vi "OEE_SCREEN_2_line_performance_into_cluster.vi"(6 "SCREEN_2":T1={"header_part_no"="-", "header_customer"="-", "performance_percentage"="-", "performance_target"="-", "performance_actual"="-", "performance_header"="PERFORMANCE", "performance_target_header"="TARGET", "performance_actual_header"="ACTUAL", "screen_2_header"=""}, 11 "hourly_ok_count":string[][](array[string])) -> (4 "SCREEN_2":T1={"header_part_no"="-", "header_customer"="-", "performance_percentage"="-", "performance_target"="-", "performance_actual"="-", "performance_header"="PERFORMANCE", "performance_target_header"="TARGET", "performance_actual_header"="ACTUAL", "screen_2_header"=""})   [LabVIEW 2019]
uses:
  typedef/SCREEN_2.ctl
  FGV/SQL_raw_data/FGV_OEE_SQL_raw_data.ctl
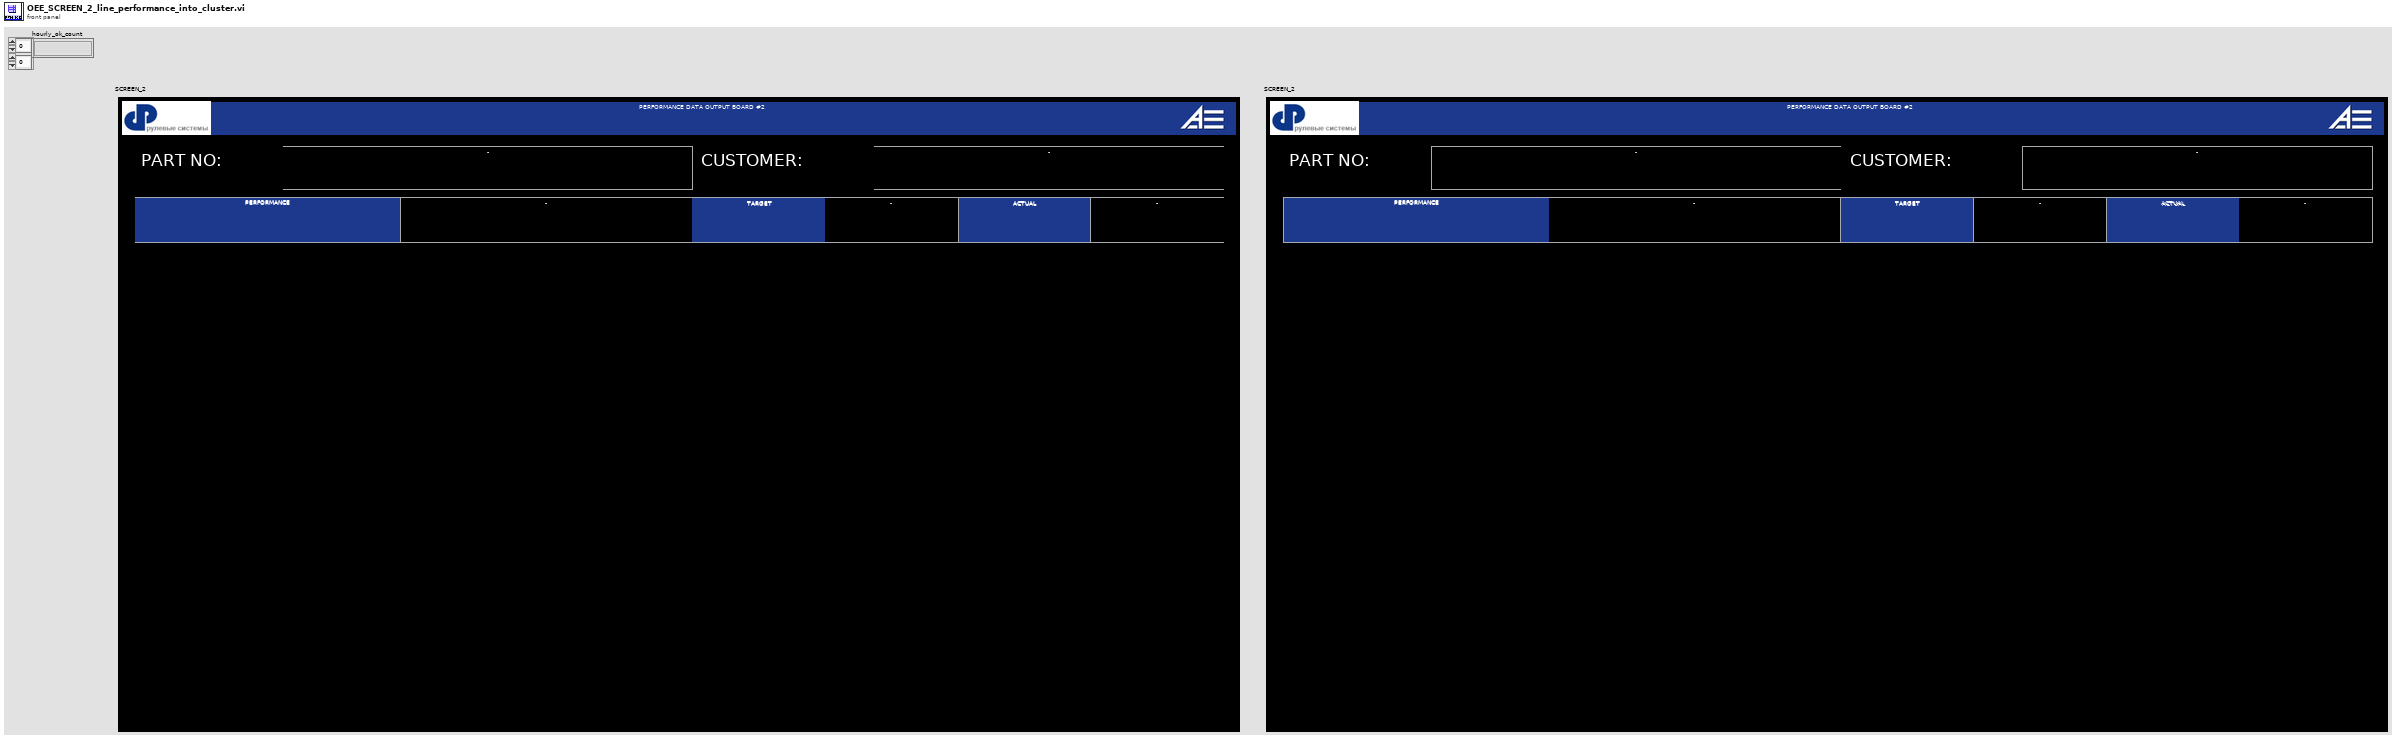
[diagram p1: front panel]
types:
  T1 = typedef "SCREEN_2.ctl" = cluster{"header_part_no":string, "header_customer":string, "performance_percentage":string, "performance_target":string, "performance_actual":string, "performance_header":string, "performance_target_header":string, "performance_actual_header":string, "screen_2_header":string}
  T2 = typedef "FGV_OEE_SQL_raw_data.ctl" = enum16{"initialize", "set_reference_name", "set_timestamp", "set_OK_NOK_count", "set_config_info", "set_pace", "set_availability", "set_hourly_ok_count", "set_targets", "get_all_info"}
  T3 = typedef "OEE_SQL_raw_data.ctl" = cluster{"reference_name":string, "data_timestamp":timestamp, "OK_NOK_count":string[][], "config_info":string[], "pace":string[][], "availability":string[], "hourly_ok_count":string[][], "shift_number":i8, "shift_start":i8, "shift_end":i8, "TAKT":u16, "FTTH_target":u16, "BOTTLENECK_station":string, "targets_hourly":u16[], "target_shift":u16}
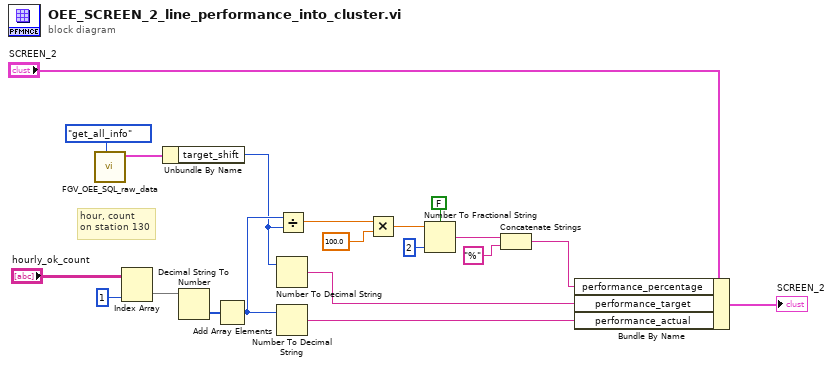
[diagram p0: block diagram]
diagram:
  # "hour, count\non station 130"
  n1 = call "FGV_OEE_SQL_raw_data.vi"("options"=FGV_OEE_SQL_raw_data."get_all_info") -> ("SQL_raw_data_out"=w12:T3)  [unwired: 9 in, 1 out]
  n2 = Index Array(array="hourly_ok_count", index (col)=1 ("index")) -> (element=w16:string[])  [unwired: 1 in]
  n3 = Unbundle By Name(w12) -> ("target_shift"=w9:u16)
  n4 = Decimal String To Number(string=w16) -> (number=w15:i32[])  [unwired: 2 in, 1 out]
  n5 = Add Array Elements(numeric array=w15) -> (sum=w10:i32)
  n6 = Number To Decimal String(number=w9) -> (decimal integer string=w11:string)  [unwired: 1 in]
  n7 = Number To Decimal String(number=w10) -> (decimal integer string=w14:string)  [unwired: 1 in]
  n8 = Divide(x=w10, y=w9) -> (x/y=w8:dbl)
  n9 = Multiply(x=w8, y=100.0) -> (x*y=w2:dbl)
  n10 = Number To Fractional String(use system decimal point (T)=FALSE, number=w2, precision (6)=i16 2) -> (F-format string=w4:string)  [unwired: 1 in]
  n11 = Concatenate Strings(w4, "%" ("string")) -> (w1:string)
  n12 = Bundle By Name(cluster="SCREEN_2", "performance_percentage"=w1, "performance_target"=w11, "performance_actual"=w14) -> (→"SCREEN_2":T1)
